vi "Shift.vi"(8 "error in":errorcluster) -> (0 "error out":errorcluster)   [LabVIEW 2015]
uses:
  Control Button/Save.ctl
  Control Button/Exit.ctl
  <vilib>/addons/database/Connection.llb/DB Tools Open Connec (String).vi
  <vilib>/addons/database/_DB Variant To Data/Database Variant To Data.xnode
  <vilib>/addons/database/NI_Database_API.lvlib
panel:
  out "error out 2":errorcluster
  out "error out":errorcluster
  out "Shift":string="B"
  in  "To-C":timestamp=timestamp(3526421399 s since 1904-01-01) format="%<%H:%M:%S\n%d/%m/%Y>T"
  in  "From-C":timestamp=timestamp(3526482600 s since 1904-01-01) format="%<%H:%M:%S\n%d/%m/%Y>T"
  in  "To-B":timestamp=timestamp(3526482599 s since 1904-01-01) format="%<%H:%M:%S\n%d/%m/%Y>T"
  in  "From-B":timestamp=timestamp(3526452000 s since 1904-01-01) format="%<%H:%M:%S\n%d/%m/%Y>T"
  in  "To-A":timestamp=timestamp(3526451999 s since 1904-01-01) format="%<%H:%M:%S\n%d/%m/%Y>T"
  in  "From-A":timestamp=timestamp(3526594200 s since 1904-01-01) format="%<%H:%M:%S\n%d/%m/%Y>T"
  in  "Exit":T1
  in  "Save":T2
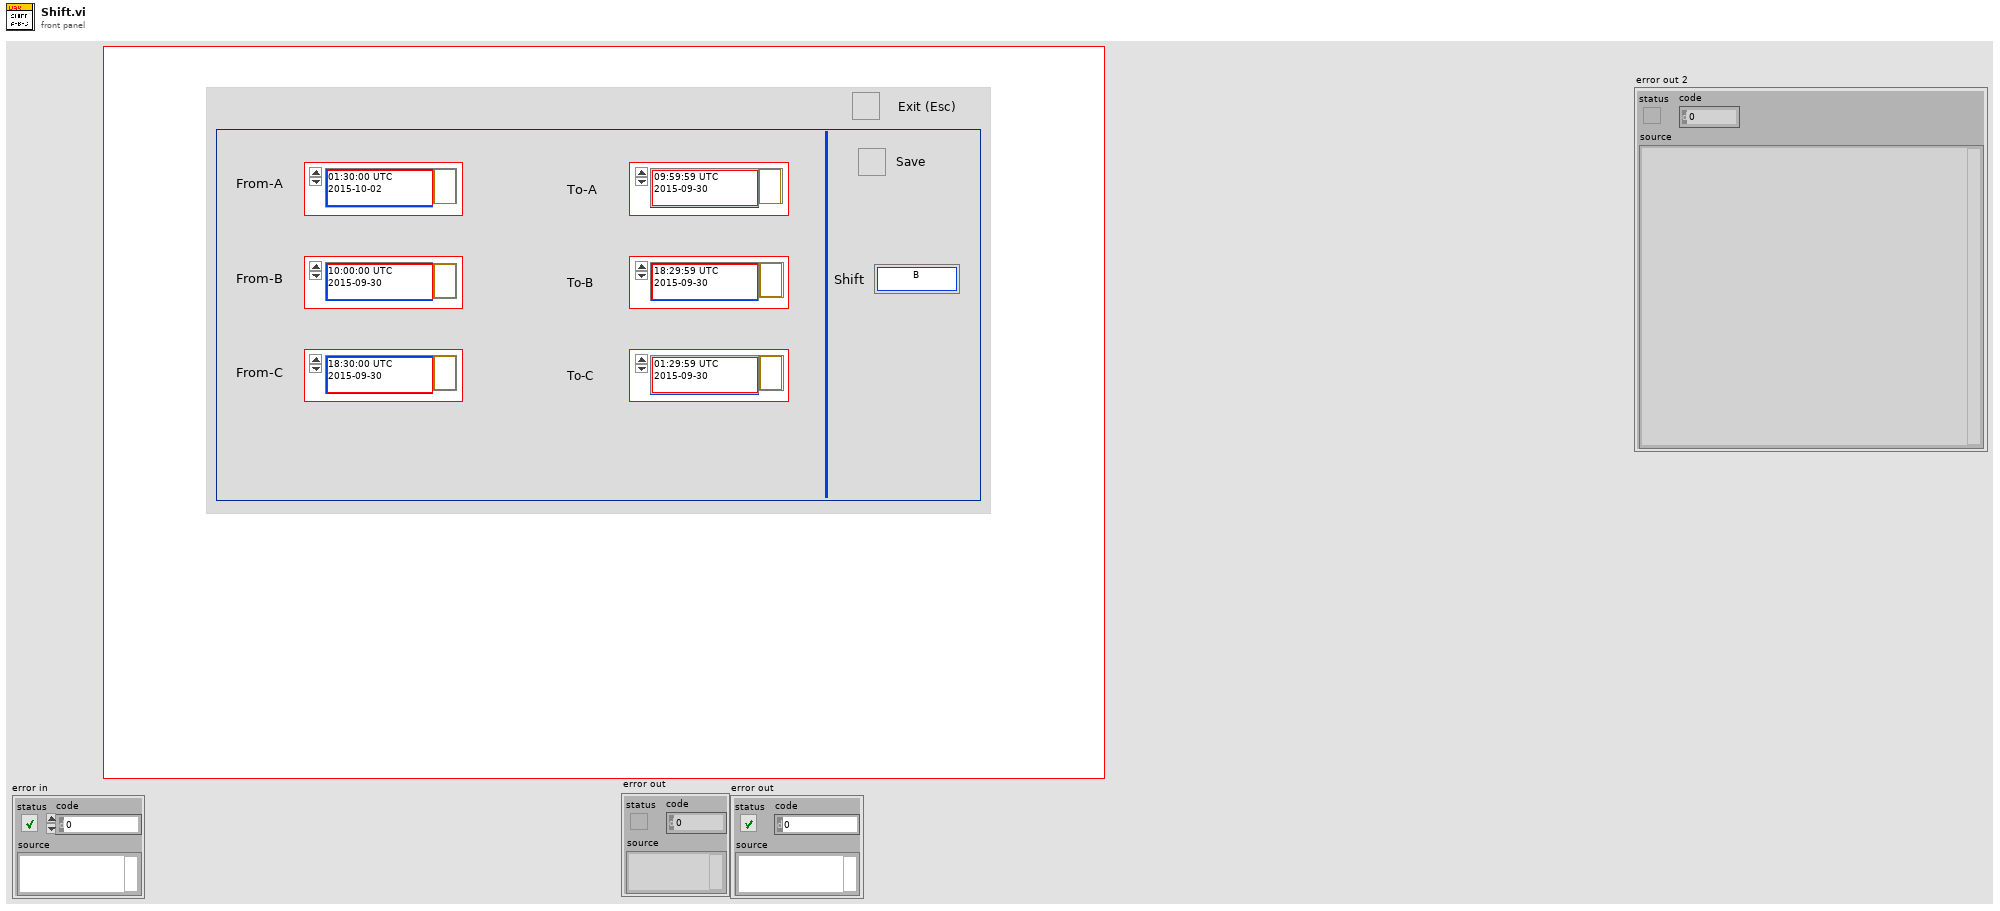
[diagram p1: front panel]
types:
  T1 = typedef "Exit.ctl" = bool
  T2 = typedef "Save.ctl" = bool
  T3 = cluster{"To-A":timestamp, "From-A":timestamp, "From-B":timestamp, "To-B":timestamp, "From-C":timestamp, "To-C":timestamp, "Shift":string}[]
  T4 = cluster{"To-A":timestamp, "From-A":timestamp, "From-B":timestamp, "To-B":timestamp, "From-C":timestamp, "To-C":timestamp, "Shift":string}
  T5 = typedef "NI_Database_API.lvlib/Conn ObjectReference.ctl" = refnum<k1>
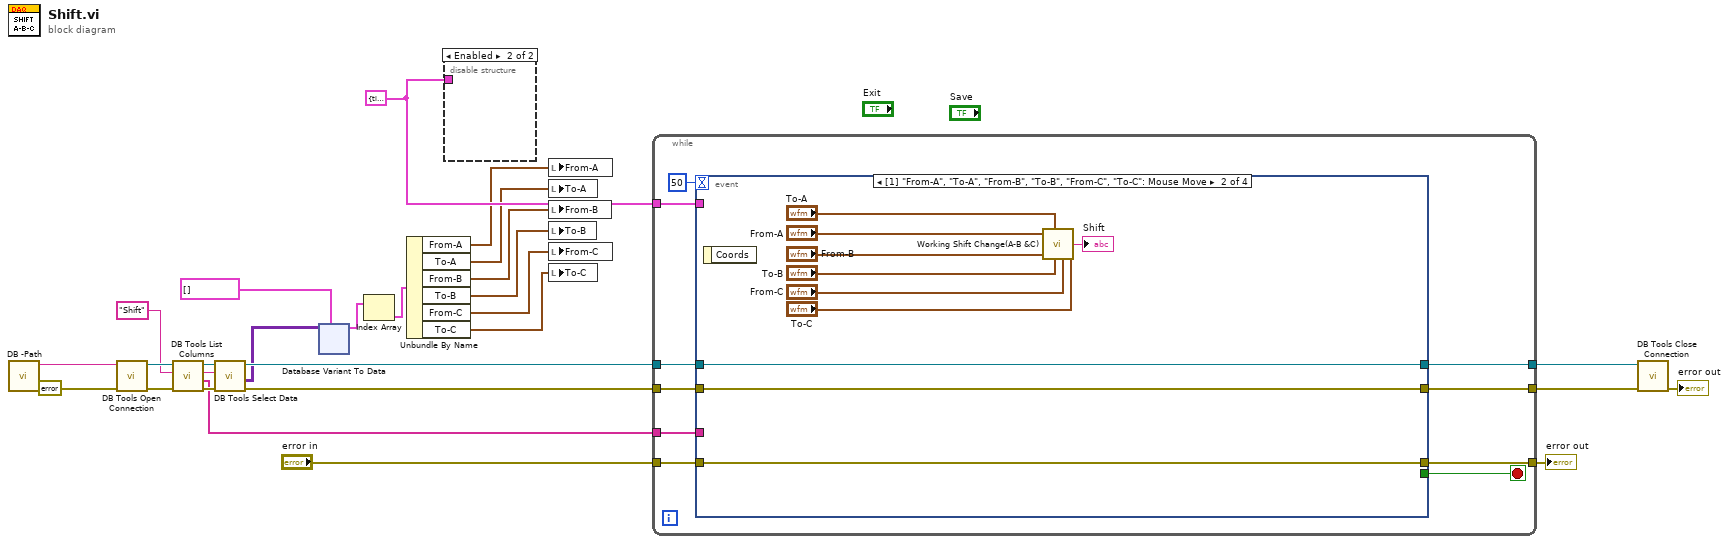
[diagram p0: block diagram]
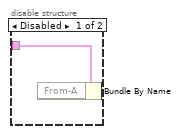
[diagram p2: hidden frame]
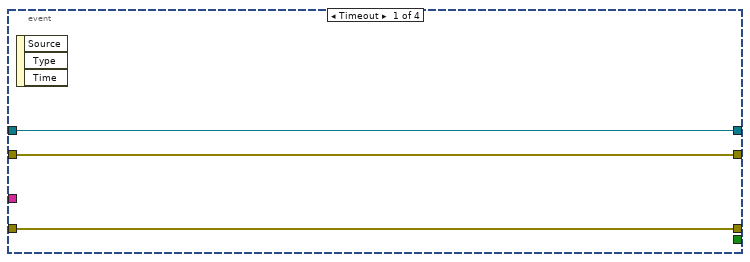
[diagram p3: hidden frame]
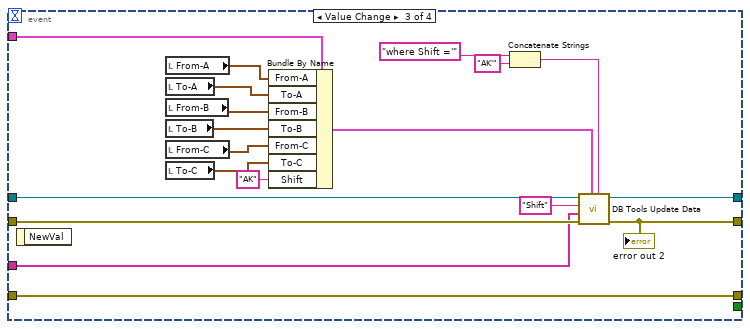
[diagram p4: hidden frame]
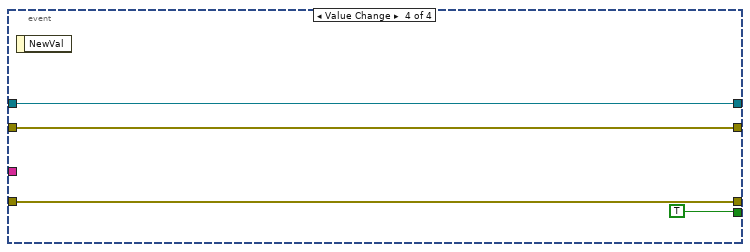
[diagram p5: hidden frame]
diagram:
  w16 = "Shift" ("table")
  w23 = T4 {"To-A"=timestamp(3526451999 s since 1904-01-01), "From-A"=timestamp(3526594200 s since 1904-01-01), "From-B"=timestamp(3526452000 s since 1904-01-01), "To-B"=timestamp(3526482599 s since 1904-01-01), "From-C"=timestamp(3526482600 s since 1904-01-01), "To-C"=timestamp(3526421399 s since 1904-01-01), "Shift"=""} ("Cluster")
  n1 = call "DB -Path.vi"() -> ("String"=w26:string)  [unwired: 11 in]
  n2 = call-poly <vilib>:"DB Tools Open Connection.vi"("error in (no error)"=errorcluster {"status"=FALSE, "code"=0, "source"=""}, "connection information"=w26) -> ("error out"=w17:errorcluster, "connection reference"=w18:T5)  [unwired: 6 in]
  n3 = call <vilib>:"DB Tools List Columns.vi"("error in (no error)"=w17, "table"=w16, "connection reference"=w18) -> ("error out"=w14:errorcluster, "columns"=w13:string[], "connection reference out"=w15:T5)  [unwired: 1 in, 1 out]
  n4 = call <vilib>:"DB Tools Select Data.vi"("error in (no error)"=w14, "table"=w16, "connection reference"=w15) -> ("error out"=w24:errorcluster, "data"=w3:variant[][], "connection reference out"=w25:T5)  [unwired: 3 in]
  n5 = xnode "Database Variant To Data"("database variant"=w3, "type"=T3 []) -> ("data"=w11:T3)  [unwired: 1 in, 1 out]
  n6 = Index Array(array=w11) -> (element=w10:T4)  [unwired: 1 in]
  n7 = Unbundle By Name(w10) -> ("From-A"=w9:timestamp, "To-A"=w8:timestamp, "From-B"=w7:timestamp, "To-B"=w6:timestamp, "From-C"=w5:timestamp, "To-C"=w4:timestamp)
  n8 = disable-structure shown="Enabled" {
    disable-tunnel: w23 -> [w27 _]
    frame Disabled {
      n9 = Bundle By Name(cluster=w27) -> ()  [unwired: 1 in, 1 out]
    }
    frame Enabled {
    }
  }
  n10 = local write "From-A"(w9) -> ()
  n11 = local write "To-A"(w8) -> ()
  n12 = local write "From-B"(w7) -> ()
  n13 = local write "To-B"(w6) -> ()
  n14 = local write "From-C"(w5) -> ()
  n15 = local write "To-C"(w4) -> ()
  n16 = while {
    tunnel: w25 -> [w36]
    tunnel: w24 -> [w35]
    tunnel: [w34] -> w22
    tunnel: [w33] -> w21
    tunnel: w23 -> [w32]
    tunnel: w13 -> [w31]
    tunnel: "error in" -> [w30]
    tunnel: [w29] -> w1
    stop <- w37 stop-if-true
    n17 = event shown="[1] \"From-A\", \"To-A\", \"From-B\", \"To-B\", \"From-C\", \"To-C\": Mouse Move" {
      selector: _ -> [_ _ _ _]
      dyn-events: _ -> [_ _ _ _]
      timeout: 50 -> [_ _ _ _]
      tunnel: [_ _ _ TRUE] -> w37
      tunnel: w36 -> [w39 w43 w66 w71]
      tunnel: w35 -> [w38 w42 w65 w70]
      tunnel: [w39 w43 w68 w71] -> w34
      tunnel: [w38 w42 w67 w70] -> w33
      tunnel: w32 -> [_ _ w64 _]
      tunnel: w31 -> [_ _ w52 _]
      tunnel: w30 -> [w40 w41 w51 w72]
      tunnel: [w40 w41 w51 w72] -> w29
      event Timeout {
        n18 = event-data() -> ()  [unwired: 1 in, 3 out]
      }
      event "From-A", "To-A", "From-B", "To-B", "From-C", "To-C": Mouse Move {
        n19 = event-data() -> ()  [unwired: 1 in, 1 out]
        n20 = call "Working Shift Change(A-B &C).vi"("From-A"="From-A", "To-A"="To-A", "From-B"="From-B", "To-B"="To-B", "From-C"="From-C", "To-C"="To-C") -> ("Shift Change"=→"Shift":string)  [unwired: 3 in]
      }
      event Value Change {
        n21 = event-data() -> ()  [unwired: 1 in, 1 out]
        n22 = local read "From-A"() -> (w63:timestamp)
        n23 = local read "To-A"() -> (w62:timestamp)
        n24 = local read "From-B"() -> (w61:timestamp)
        n25 = local read "To-B"() -> (w60:timestamp)
        n26 = local read "From-C"() -> (w59:timestamp)
        n27 = local read "To-C"() -> (w58:timestamp)
        n28 = Bundle By Name(cluster=w64, "From-A"=w63, "To-A"=w62, "From-B"=w61, "To-B"=w60, "From-C"=w59, "To-C"=w58, "Shift"="AK") -> (w69:T4)
        n29 = Concatenate Strings("where Shift ='" ("string"), "AK'" ("string")) -> (w53:string)
        n30 = call <vilib>:"DB Tools Update Data.vi"("condition"=w53, "data"=w69, "error in (no error)"=w65, "columns"=w52, "table"="Shift", "connection reference"=w66) -> ("error out"=w67:errorcluster, "connection reference out"=w68:T5)  [unwired: 4 in]
        "error out 2" <- w67
      }
      event Value Change {
        n31 = event-data() -> ()  [unwired: 1 in, 1 out]
      }
    }
  }
  "error out" <- w1
  n32 = call <vilib>:"DB Tools Close Connection.vi"("error in (no error)"=w21, "connection reference"=w22) -> ("error out"=→"error out":errorcluster)  [unwired: 5 in]
